vi "test_UDP Read.vi"(8 "error in (no error)":errorcluster, 11 "TestCase in":refnum<class "Instrument Addon Ethernet Protocol Unit Tests.lvclass">) -> (0 "error out":errorcluster, 3 "TestCase out":refnum<class "Instrument Addon Ethernet Protocol Unit Tests.lvclass">)   [LabVIEW 2023, in "Instrument Addon Ethernet Protocol Unit Tests.lvclass"]
uses:
  Instrument Addon Ethernet Protocol Unit Tests.lvclass
  <vilib>/addons/_JKI Toolkits/VI Tester/TestCase.llb/TestCase.lvclass
  UDP/UDP.lvclass
  Listener/Listener.lvclass
  Listener/ListenerClassControls/Operation.ctl
  Protocol Parent/Methods/Read Parameter.ctl
  Protocol Parent/Protocol Parent.lvclass
  Constants.vi
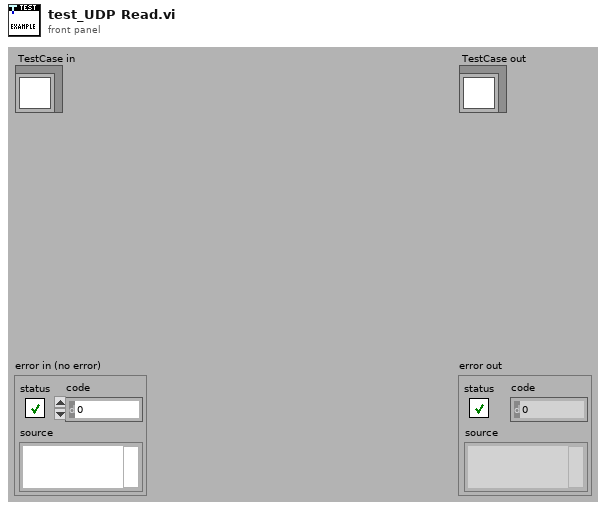
[diagram p1: front panel]
types:
  T1 = typedef "Protocols.lvlib/Protocol Parent.lvclass/Read Parameter.ctl" = cluster{"Wait Type":enum16{"Byte Count", "Wait sec"}, "Wait Value":dbl}
  T2 = typedef "Listener.lvclass/Operation.ctl" = enum16{"Read", "Write"}
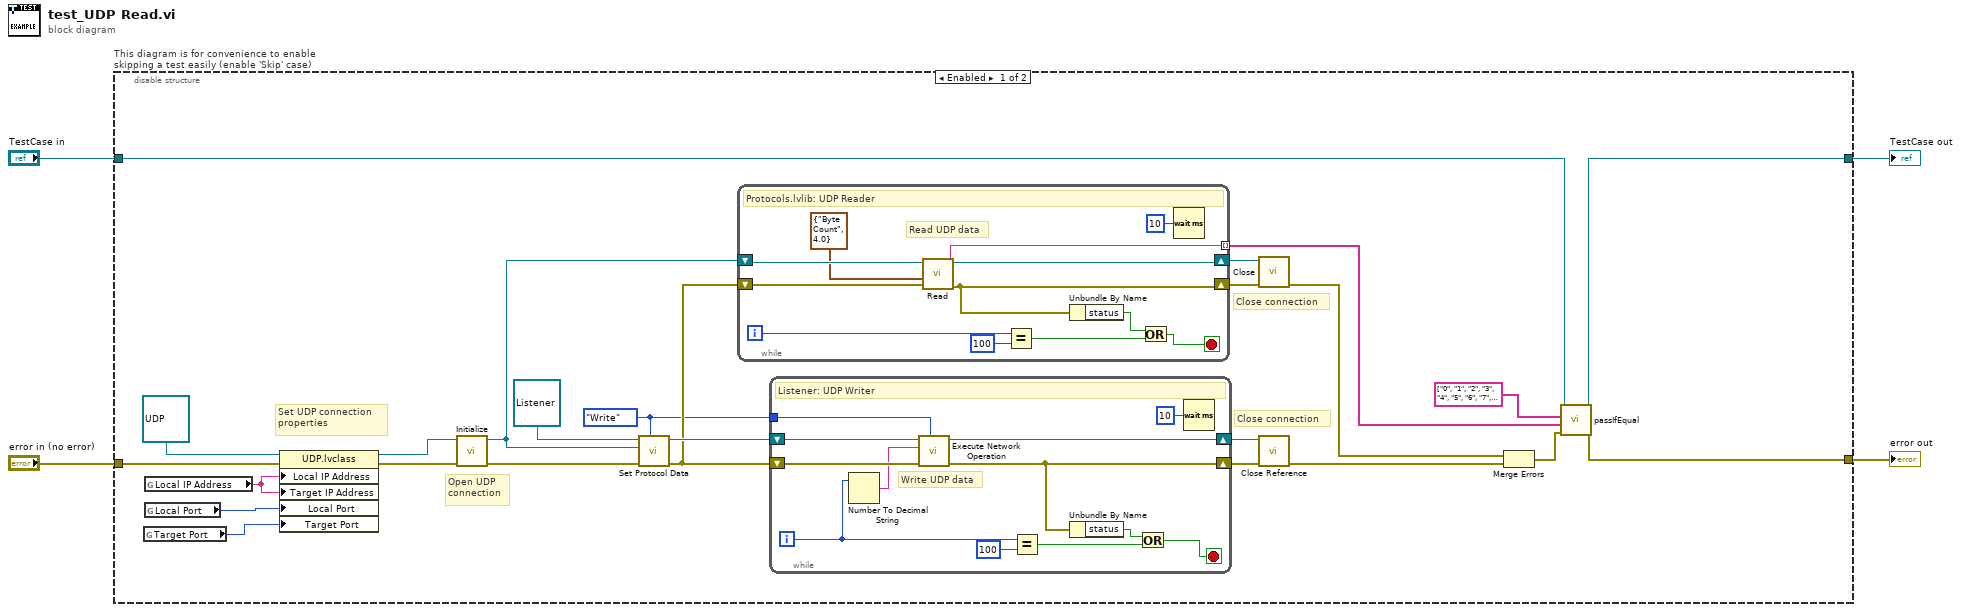
[diagram p0: block diagram]
diagram:
  n1 = disable-structure "This diagram is for convenience to enable skipping a test easily (enable 'Skip' case)" shown="Enabled" {
    disable-tunnel: "TestCase in" -> [w29 w57]
    disable-tunnel: [w28 w55] -> w1
    disable-tunnel: [w27 w56] -> w3
    disable-tunnel: "error in (no error)" -> [w25 w54]
    frame Enabled {
      w5 = Operation."Write" ("Operation")
      # "Close connection"
      # "Close connection"
      # "Open UDP \nconnection"
      # "Set UDP connection \nproperties"
      n2 = global read "Constants.vi" "Target Port"() -> (w6:u16)
      n3 = global read "Constants.vi" "Local IP Address"() -> (w8:string)
      n4 = global read "Constants.vi" "Local Port"() -> (w7:u16)
      n5 = property class="UDP.lvclass"(reference=refnum<class "UDP.lvclass"> refnum ("Protocols.lvlib:UDP.lvclass"), error in=w25, "Local IP Address"=w8, "Target IP Address"=w8, "Local Port"=w7, "Target Port"=w6) -> (reference out=w24:refnum<class "UDP.lvclass">, error out=w23:errorcluster)
      n6 = call-dynamic "Initialize.vi"("error in (no error)"=w23, "UDP in"=w24) -> ("error out"=w22:errorcluster, "UDP out"=w19:refnum<class "UDP.lvclass">)  [unwired: 8 in]
      n7 = call "Set Protocol Data.vi"("Operation"=w5, "error in (no error)"=w22, "Protocols.lvlib:Protocol Parent.lvclass"=w19, "Listener In.lvclass"=refnum<class "Listener.lvclass"> refnum ("Listener.lvclass")) -> ("error out"=w18:errorcluster, "Listener Out.lvclass"=w20:refnum<class "Listener.lvclass">)  [unwired: 6 in]
      n8 = while {
        shift-right: [w46] -> w14
        shift-left: w18 -> [w44]
        shift-right: [w45] -> w13
        shift-left: w19 -> [w53]
        tunnel: [w43] -> w17 mode=indexing
        i -> [w51]
        stop <- w47 stop-if-true
        # "Read UDP data"
        # "Protocols.lvlib: UDP Reader"
        n9 = call-dynamic "Read.vi"("error in (no error)"=w44, "Variant"=T1 {"Wait Type"=enum."Byte Count", "Wait Value"=4.0} ("Read Parameter"), "UDP in"=w53) -> ("error out"=w46:errorcluster, "String"=w43:string, "UDP out"=w45:refnum<class "UDP.lvclass">)  [unwired: 6 in]
        n10 = Equal?(x=w51, y=100) -> (x = y?=w49:bool)
        n11 = Unbundle By Name(w46) -> ("status"=w48:bool)
        n12 = Or(x=w48, y=w49) -> (x .or. y?=w47:bool)
        n13 = Wait (ms)(milliseconds to wait=u32 10) -> ()  [unwired: 1 out]
      }
      n14 = while {
        shift-right: [w38] -> w10
        shift-left: w20 -> [w40]
        shift-right: [w35] -> w11
        shift-left: w18 -> [w41]
        tunnel: w5 -> [w30]
        i -> [w32]
        stop <- w33 stop-if-true
        # "Write UDP data"
        # "Listener: UDP Writer"
        n15 = Number To Decimal String(number=w32) -> (decimal integer string=w31:string)  [unwired: 1 in]
        n16 = call "Execute Network Operation.vi"("Operation"=w30, "error in (no error)"=w41, "Message"=w31, "Listener In.lvclass"=w40) -> ("error out"=w35:errorcluster, "Listener Out.lvclass"=w38:refnum<class "Listener.lvclass">)  [unwired: 6 in]
        n17 = Equal?(x=w32, y=100) -> (x = y?=w36:bool)
        n18 = Unbundle By Name(w35) -> ("status"=w34:bool)
        n19 = Or(x=w34, y=w36) -> (x .or. y?=w33:bool)
        n20 = Wait (ms)(milliseconds to wait=u32 10) -> ()  [unwired: 1 out]
      }
      n21 = call-dynamic "Close.vi"("error in (no error)"=w14, "UDP in"=w13) -> ("error out"=w12:errorcluster)  [unwired: 8 in, 1 out]
      n22 = call "Close Reference.vi"("error in (no error)"=w11, "Listener In.lvclass"=w10) -> ("error out"=w9:errorcluster)  [unwired: 8 in, 1 out]
      n23 = Merge Errors(w12, w9) -> (w16:errorcluster)
      n24 = call-dynamic "passIfEqual.vi"("error in (no error)"=w16, "y"=w17, "x"=string[] ["0", "1", "2", "3", "4", "5", "6", "7", "8", "9", "10", "11", "12", "13", "14", "15", "16", "17", "18", "19", "20", "21", "22", "23", "24", "25", "26", "27", "28", "29", "30", "31", "32", "33", "34", "35", "36", "37", "38", "39", "40", "41", "42", "43", "44", "45", "46", "47", "48", "49", "50", "51", "52", "53", "54", "55", "56", "57", "58", "59", "60", "61", "62", "63", "64", "65", "66", "67", "68", "69", "70", "71", "72", "73", "74", "75", "76", "77", "78", "79", "80", "81", "82", "83", "84", "85", "86", "87", "88", "89", "90", "91", "92", "93", "94", "95", "96", "97", "98", "99", "100"] ("Array"), "TestCase in"=w29) -> ("error out"=w27:errorcluster, "TestCase out"=w28:refnum<class "Instrument Addon Ethernet Protocol Unit Tests.lvclass">)  [unwired: 6 in]
    }
    frame Disabled {
      # "skip test result while test is under development"
      n25 = call <vilib>:"skip.vi"("error in (no error)"=w54, "TestCase in"=w57) -> ("error out"=w56:errorcluster, "TestCase out"=w55:refnum<class "Instrument Addon Ethernet Protocol Unit Tests.lvclass">)  [unwired: 8 in]
    }
  }
  "error out" <- w3
  "TestCase out" <- w1
